vi "Write Project Ref.vi"(8 "error in (no error)":errorcluster, 10 "Project Ref":refnum<vi>, 11 "Project in":refnum<class "Project.lvclass">) -> (0 "error out":errorcluster, 3 "Project out":refnum<class "Project.lvclass">)   [LabVIEW 2019, in "Panther Dashboard.lvlib" / "Project.lvclass"]
uses:
  Project.lvclass
  Project.lvclass/Project.ctl
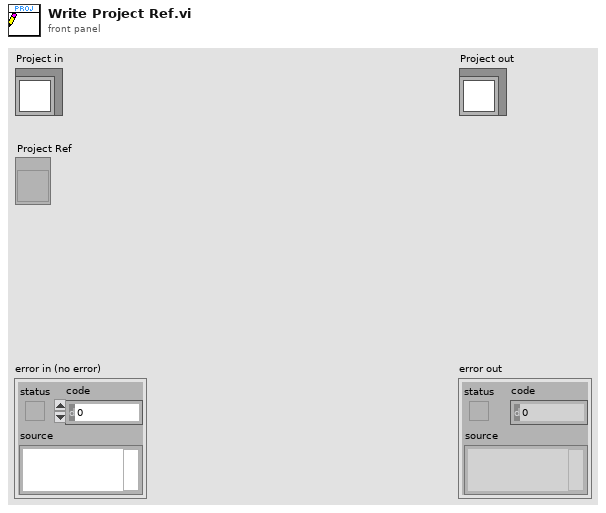
[diagram p1: front panel]
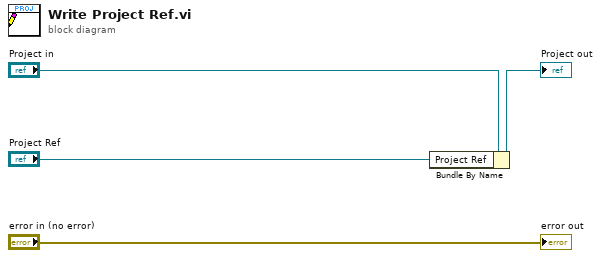
[diagram p0: block diagram]
diagram:
  n1 = Bundle By Name(cluster="Project in", "Project Ref"="Project Ref") -> (→"Project out":refnum<class "Project.lvclass">)
  "error out" <- "error in (no error)"
